vi "SetMailSailPos.vi"(8 "error in (no error)":errorcluster, 10 "MainSailPos":dbl, 11 "RealSail in":refnum<class "RealSail.lvclass">) -> (0 "error out":errorcluster, 3 "RealSail out":refnum<class "RealSail.lvclass">)   [LabVIEW 2013, in "RealSail.lvclass"]
uses:
  RealSail.lvclass
  AbstractSail/AbstractSail.lvclass
  <vilib>/rvi/interface/nirviReadWriteControl/nirviReadWriteControl.xnode
  <vilib>/rvi/interface/Simulation/niFpgaSimulationCallBeginRW.vi
  <vilib>/rvi/errors/niLvFpgaAdjustHostInterfaceError.vi
panel:
  out "FPGA VI Reference Out":refnum<k20>
  in  "FPGA VI Reference In":refnum<k20>
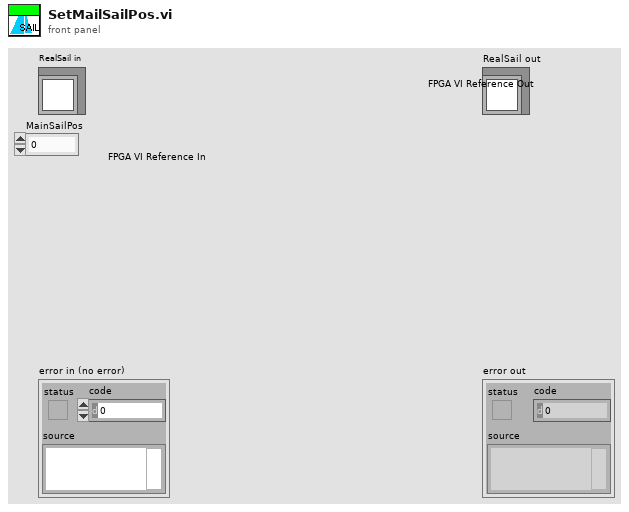
[diagram p1: front panel]
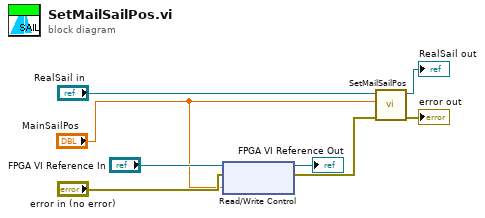
[diagram p0: block diagram]
diagram:
  n1 = xnode "Read/Write Control"("FPGA VI Reference In"="FPGA VI Reference In", "error in"="error in (no error)", "Unselected"="MainSailPos") -> ("FPGA VI Reference Out"=→"FPGA VI Reference Out":refnum<k20>, "error out"=w2:errorcluster)
  n2 = call-parent "SetMailSailPos.vi"("error in (no error)"=w2, "MainSailPos"="MainSailPos", "AbstractSail in"="RealSail in") -> ("error out"=→"error out":errorcluster, "AbstractSail out"=→"RealSail out":refnum<class "RealSail.lvclass">)  [unwired: 7 in]
